vi "WSVCAP SHL Host TL Tester.vi"(0 "FPGA":T1) -> ()   [LabVIEW 2017]
uses:
  Type Defs/WSVCAP SHL DUT Number Enum.ctl
  <vilib>/userdefined/High Color/nirio_resource_hc.ctl
  Type Defs/WSVCAP SHL FPGA Enum.ctl
  Type Defs/WSVCAP SHL Tester System Cluster.ctl
  Type Defs/WSVCAP SHL I2C DUT Mask Mode Enum.ctl
panel:
  in  "Cap DAC":u8=144 caption="B Data In" format="0x%02x"
  in  "Set Cap DAC":bool
  in  "CP 35V":bool
  in  "CP 23.75V":bool
  in  "DVA On":bool
  in  "DVA Off":bool
  in  "CP 44V":bool
  in  "CP 40.25V":bool
  in  "Read Data DUT CMD":string caption="Read Data Out"
  in  "Read DUT":bool
  in  "CP On":bool
  in  "CP Off":bool
  in  "Write DUT":bool
  in  "Write Data DUT":string caption="Write Data Out"
  out "Read Data DUT Out":string caption="Data In"
  in  "Stop RFFE Cycle":bool
  in  "Start RFFE Cycle":bool
  in  "Command":string[](array[string])=["0703010F0F0F0F", "07030100000000"]
  in  "Post CMd Delay":dbl[](array[numeric])=[1.2e-05, 5.4e-05] min=0.0 max=0.5 format="%#.0p s"
  in  "Number of Commands":u32=2 min=1 max=4 step=1
  out "Cycle Count":u64=2 min=1 max=4 step=1
  in  "Monitor":bool
  out "AD7747 Values":string[][](table)
  in  "Mode":enum32{"All", "Single"}(radio)
  in  "RFFE Slave Address":u8=144 caption="Slave Address" format="0x%02x"
  out "Activity Log":string
  out "Simulate FPGA":bool
  out "Online":bool
  out "FPGA Resource":T2
  out "Status":string
  out "Busy":bool
  in  "I2C Bytes to Read":u8=1 caption="Bytes" min=1 max=4 step=1
  in  "Exit":bool
  out "Read Data I2C":u8[](array[numeric]) caption="Data In" format="0x%02x"
  in  "Read Reg I2C":u8 caption="Register" format="0x%02x"
  in  "Read I2C":bool
  in  "DUT":T3
  in  "Write Data I2C":u8 caption="Data Out" format="0x%02x"
  in  "Write Reg I2C":u8=144 caption="Register" format="0x%02x"
  in  "I2C Init":bool
  in  "Init Data":u8[](array[numeric])=[164, 160, 14, 33] caption="Data Out" format="0x%02x"
  in  "Init Reg":u8[](array[numeric])=[191, 7, 9, 10] caption="Register" format="0x%02x"
  in  "Write I2C":bool
  in  "I2C Slave Address":u8=144 caption="Slave Address" format="0x%02x"
  in  "RFFE Clock Rate (Hz)":dbl=1000000.0 caption="Clock Rate" format="%.1p Hz"
  in  "I2C Clock Rate (Hz)":dbl=100000.0 caption="Clock Rate" format="%.0p Hz"
  in  "Error":errorcluster
  # "WS1020 Tester"
  # "AD7747 (I2C)"
  # "C"
  # "DUT Control (RFFE)"
  # "DUT Cycling (RFFE)"
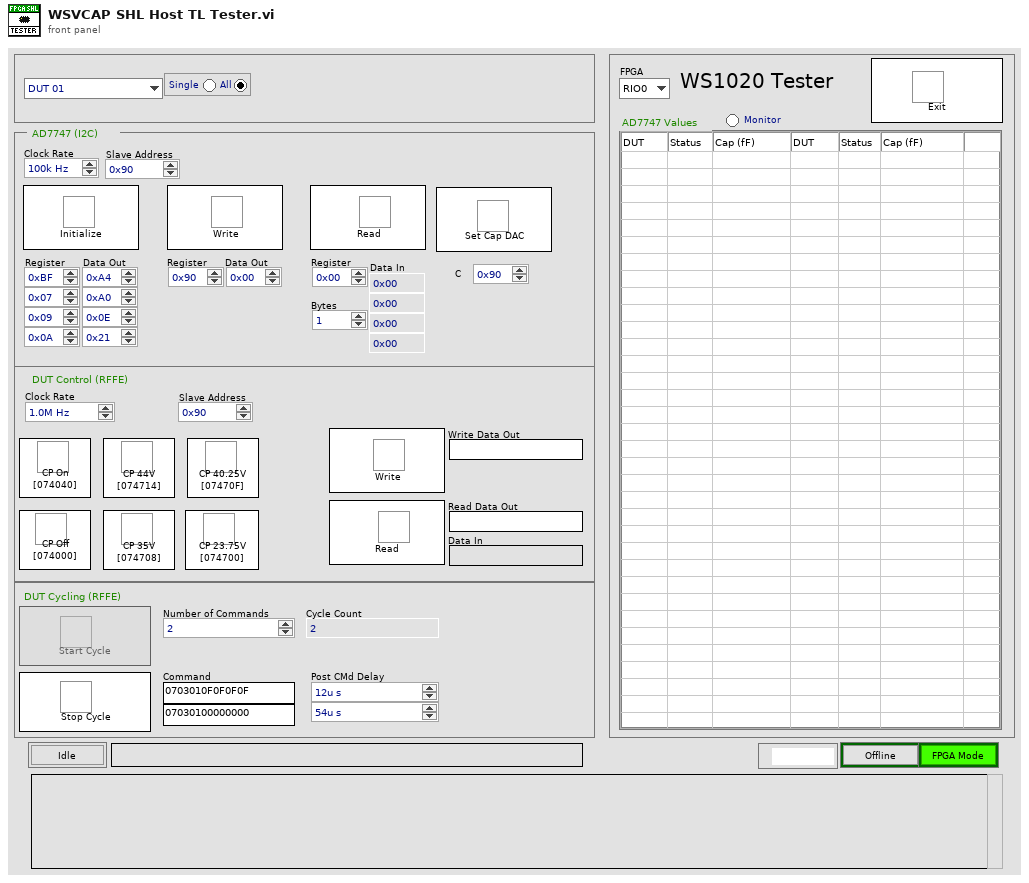
[diagram p1: front panel]
types:
  T1 = typedef "WSVCAP SHL FPGA Enum.ctl" = enum16{"RIO0", "RIO1"}
  T2 = typedef "nirio_resource_hc.ctl" = tag
  T3 = typedef "WSVCAP SHL DUT Number Enum.ctl" = enum16{"DUT 01", "DUT 02", "DUT 03", "DUT 04", "DUT 05", "DUT 06", "DUT 07", "DUT 08", "DUT 09", "DUT 10", "DUT 11", "DUT 12", "DUT 13", "DUT 14", "DUT 15", "DUT 16", "DUT 17", "DUT 18", "DUT 19", "DUT 20", "DUT 21", "DUT 22", "DUT 23", "DUT 24", "DUT 25", "DUT 26", "DUT 27", "DUT 28", "DUT 29", "DUT 30", "DUT 31", "DUT 32", "DUT 33", "DUT 34", "DUT 35", "DUT 36", "DUT 37", "DUT 38", "DUT 39", "DUT 40", "DUT 41", "DUT 42", "DUT 43", "DUT 44", "DUT 45", "DUT 46", "DUT 47", "DUT 48", "DUT 49", "DUT 50", "DUT 51", "DUT 52", "DUT 53", "DUT 54", "DUT 55", "DUT 56", "DUT 57", "DUT 58", "DUT 59", "DUT 60", "DUT 61", "DUT 62", "DUT 63", "DUT 64"}
  T4 = typedef "WSVCAP SHL Tester System Cluster.ctl" = cluster{"I2C Monitor":bool, "SPI Cyle":bool, "SPI Mode":enum32{"Write/Read", "Cycle"}, "RFFE Cyle":bool, "RFFE Mode":enum32{"Write/Read", "Cycle"}}
  T5 = typedef "WSVCAP SHL Core System Cluster.ctl" = cluster{"Settings":T6, "FPGA Resource":tag, "Online":bool, "I2C Wait Ticks":u32, "SPI Wait Ticks":u32, "RFFE Wait Ticks":u32, "FPGA VI Reference (FPGA Mode)":T7, "FPGA VI Reference (Sim Mode)":refnum<vi>}
  T6 = typedef "WSVCAP SHL I2C Settings Cluster.ctl" = cluster{"I2C Slave Address":u8, "I2C Clock Rate (Hz)":dbl, "SPI Clock Rate (Hz)":dbl, "RFFE Slave Address":u8, "RFFE Clock Rate (Hz)":dbl, "Simulate FPGA":bool, "C1 Cap DAC Default":u8, "C2 Cap DAC Default":u8, "C3 Cap DAC Default":u8, "C4 Cap DAC Default":u8}
  T7 = typedef "WSVCAP SHL FPGA Ref.ctl" = refnum<k20>
  T8 = enum8{"Enabled", "Disabled", "Disabled and Grayed Out"}
  T9 = typedef "WSVCAP SHL I2C DUT Mask Mode Enum.ctl" = enum16{"Custom", "All"}
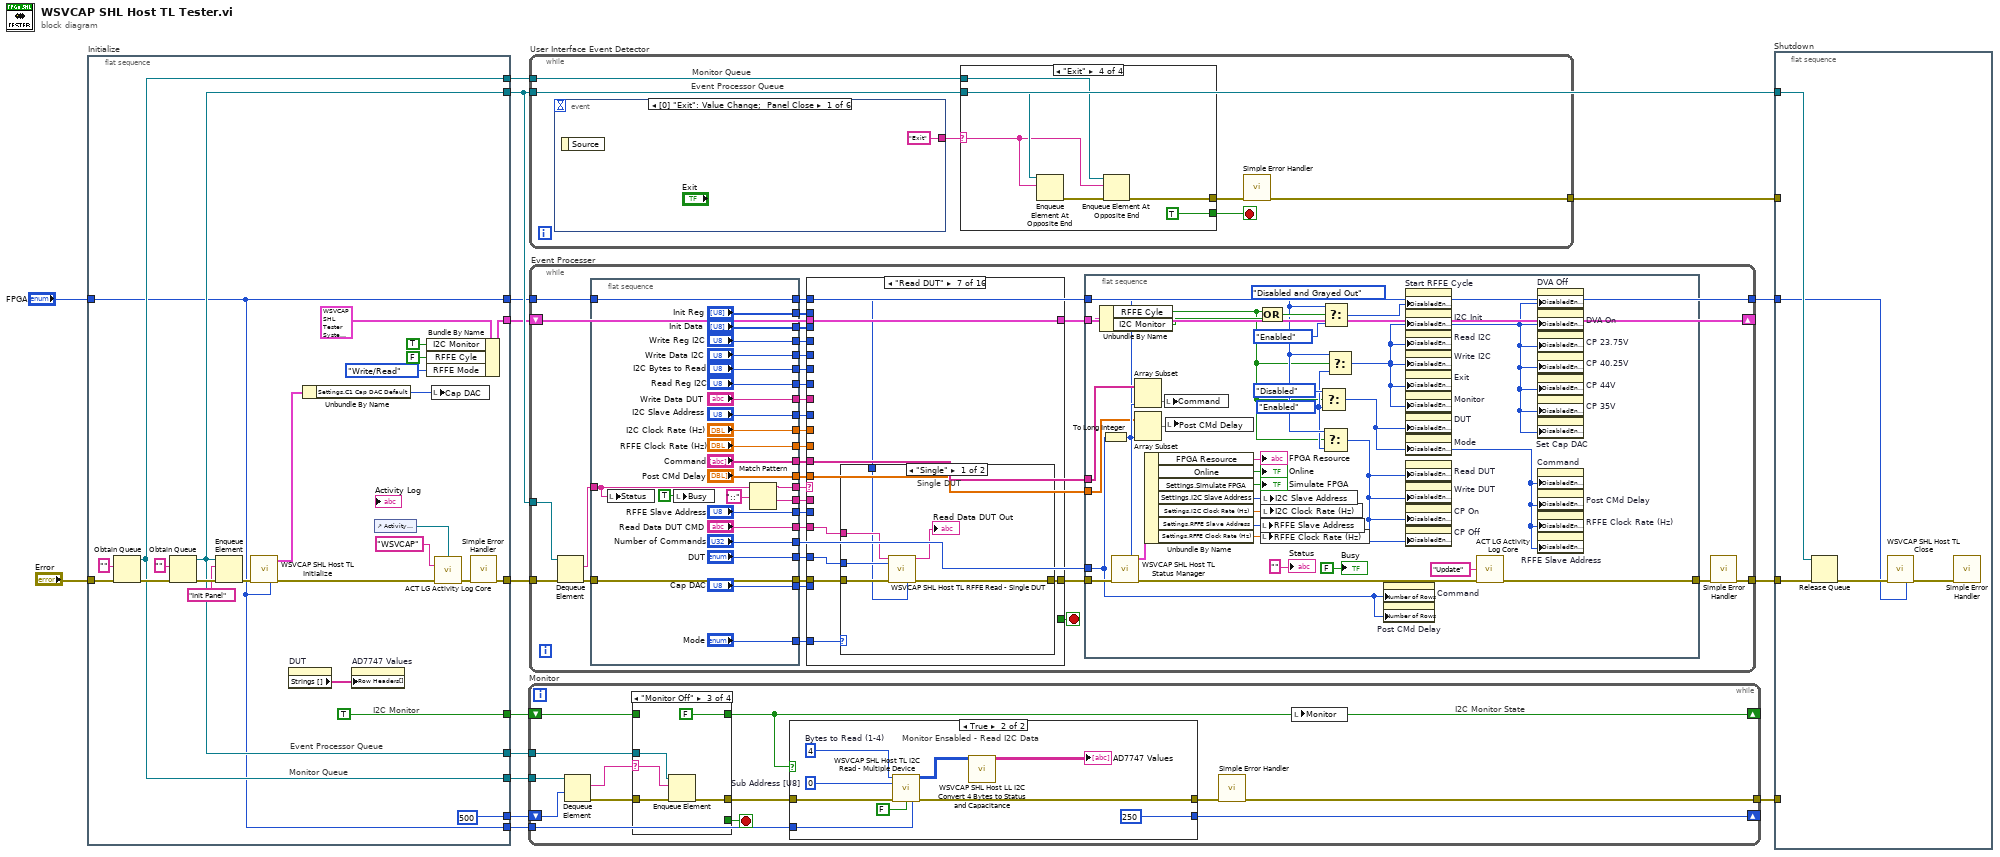
[diagram p0: block diagram]
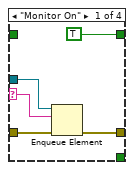
[diagram p2: hidden frame]
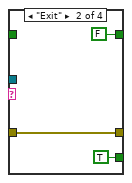
[diagram p3: hidden frame]
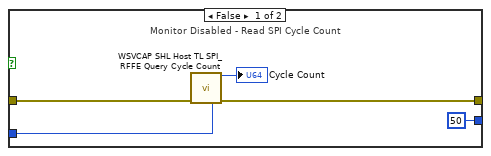
[diagram p5: hidden frame]
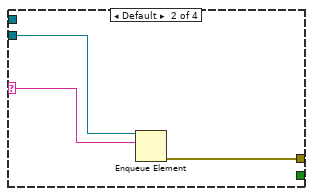
[diagram p7: hidden frame]
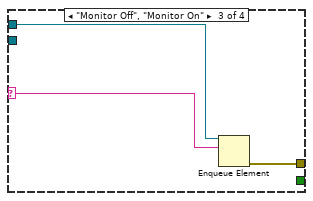
[diagram p8: hidden frame]
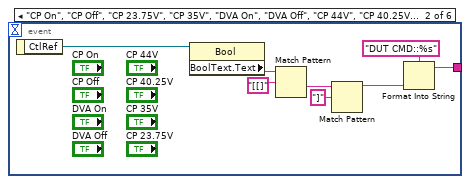
[diagram p9: hidden frame]
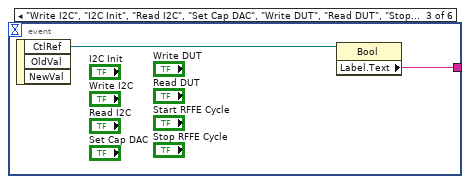
[diagram p10: hidden frame]
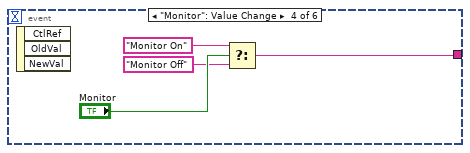
[diagram p11: hidden frame]
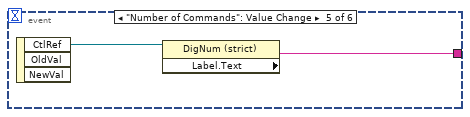
[diagram p12: hidden frame]
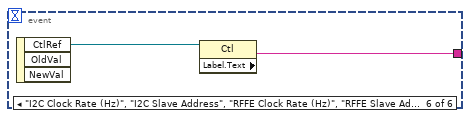
[diagram p13: hidden frame]
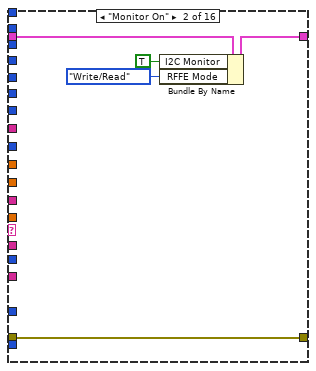
[diagram p15: hidden frame]
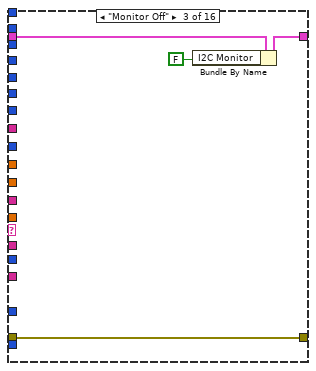
[diagram p16: hidden frame]
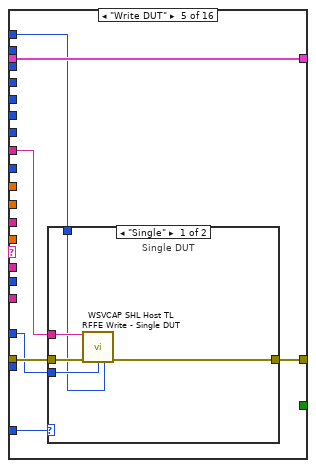
[diagram p18: hidden frame]
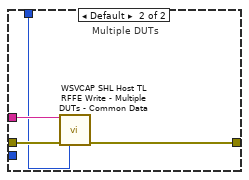
[diagram p19: hidden frame]
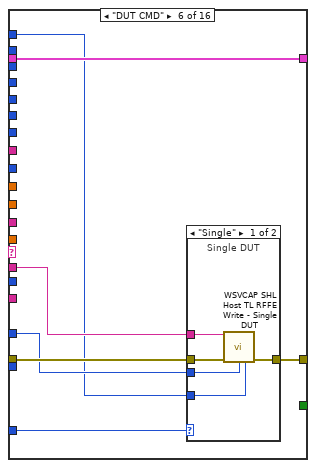
[diagram p20: hidden frame]
diagram:
  n1 = flat-sequence "Initialize" {
    tunnel: "Error" -> [w32]
    tunnel: [w30] -> w15
    tunnel: [TRUE ("Monitor")] -> w6
    tunnel: [w37] -> w11
    tunnel: [w28] -> w10
    tunnel: [w25] -> w9
    tunnel: [w30] -> w8
    tunnel: [w25] -> w7
    tunnel: [500 ("Wait Time (500ms)")] -> w5
    tunnel: "FPGA" -> [w17]
    tunnel: [w17] -> w3
    tunnel: [w17] -> w1
    frame #0 {
      # "I2C Monitor"
      # "Monitor Queue"
      # "Event Processor Queue"
      n2 = Obtain Queue(element data type="" ("name (unnamed)"), error in (no error)=w32) -> (queue out=w25:refnum<queue>, error out=w31:errorcluster)  [unwired: 3 in, 1 out]
      n3 = Obtain Queue(element data type="" ("name (unnamed)"), error in (no error)=w31) -> (queue out=w30:refnum<queue>, error out=w40:errorcluster)  [unwired: 3 in, 1 out]
      n4 = Enqueue Element(queue=w30, element="Init Panel" ("name (unnamed)"), error in (no error)=w40) -> (error out=w22:errorcluster)  [unwired: 1 in, 2 out]
      n5 = call "WSVCAP SHL Host TL Initialize.vi"("error in"=w22, "FPGA"=w17) -> ("System"=w20:T5, "error out"=w21:errorcluster)  [unwired: 12 in]
      n6 = property on="DUT" class="Enum (strict)"() -> ("Strings []"=w23:string[])  [unwired: 2 in, 2 out]
      n7 = Unbundle By Name(w20) -> ("Settings.C1 Cap DAC Default"=w19:u8)
      n8 = property on="AD7747 Values" class="Tbl (strict)"("Row Headers[]"=w23) -> ()  [unwired: 2 in, 2 out]
      n9 = control-ref of="Activity Log"() -> (w36:refnum<vi>)
      n10 = Bundle By Name(cluster=T4 {"I2C Monitor"=TRUE, "SPI Cyle"=TRUE, "SPI Mode"=enum."Write/Read", "RFFE Cyle"=FALSE, "RFFE Mode"=enum."Write/Read"}, "I2C Monitor"=TRUE, "RFFE Cyle"=FALSE ("I2C Monitor"), "RFFE Mode"=enum32{"Write/Read", "Cycle"}."Write/Read" ("SPI Mode")) -> (w28:T4)
      n11 = local write "Cap DAC"(w19) -> ()
      n12 = call "ACT LG Activity Log Core.vi"("Display Ref"=w36, "Source"="WSVCAP", "Error In (no error)"=w21) -> ("Error Out"=w38:errorcluster)  [unwired: 11 in, 1 out]
      n13 = call <vilib>:"Simple Error Handler.vi"("error in (no error)"=w38) -> ("error out"=w37:errorcluster)  [unwired: 4 in, 4 out]
    }
  }
  n14 = while "Monitor" {
    tunnel: [w46] -> w12
    shift-right: [w45] -> _
    shift-left: w6 -> [w52]
    tunnel: w9 -> [w50]
    tunnel: w8 -> [w49]
    shift-right: [w44] -> _
    shift-left: w5 -> [w43]
    tunnel: w1 -> [w42]
    stop <- w47 stop-if-true
    # "I2C Monitor State"
    n15 = Dequeue Element(queue=w50, timeout in ms (-1)=w43) -> (element=w53:string, error out=w51:errorcluster)  [unwired: 1 in, 2 out]
    n16 = case shown="\"Monitor Off\"" w53 {
      selector: w53 -> [w56 _ w64 _]
      tunnel: [TRUE FALSE FALSE w69] -> w45
      tunnel: w52 -> [_ _ _ w69]
      tunnel: w51 -> [w58 w61 w66 w68]
      tunnel: [w57 w61 w65 w68] -> w48
      tunnel: w49 -> [w55 _ w63 _]
      tunnel: [_ TRUE _ _] -> w47
      frame "Monitor On" {
        n17 = Enqueue Element(queue=w55, element=w56, error in (no error)=w58) -> (error out=w57:errorcluster)  [unwired: 1 in, 2 out]
      }
      frame "Exit" {
      }
      frame "Monitor Off" {
        n18 = Enqueue Element(queue=w63, element=w64, error in (no error)=w66) -> (error out=w65:errorcluster)  [unwired: 1 in, 2 out]
      }
      frame Default {
      }
    }
    n19 = case shown="True" w45 {
      tunnel: [w72 w78] -> w54
      tunnel: w48 -> [w73 w79]
      tunnel: [50 ("Wait Time (500ms)") 250 ("Wait Time (500ms)")] -> w44
      tunnel: w42 -> [w70 w75]
      frame False {
        # "Monitor Disabled - Read SPI Cycle Count"
        n20 = call "WSVCAP SHL Host TL SPI_RFFE Query Cycle Count.vi"("error in"=w73, "FPGA"=w70) -> ("Cycle Count"=→"Cycle Count":u64, "error out"=w72:errorcluster)  [unwired: 12 in]
      }
      frame True {
        w82 = u8 4  # Bytes to Read (1-4)
        w83 = u8 0  # Sub Address [U8]
        # "Monitor Ensabled - Read I2C Data"
        n21 = call "WSVCAP SHL Host TL I2C Read - Multiple Device.vi"("Bytes to Read (1-4)"=w82, "Sub Address [U8]"=w83, "error in"=w79, "Log (T)"=FALSE, "FPGA"=w75) -> ("C:1-64 Read Data [U8]"=w81:u8[][], "error out"=w78:errorcluster)  [unwired: 9 in]
        n22 = call "WSVCAP SHL Host LL I2C Convert 4 Bytes to Status and Capacitance.vi"("C:1-64 Read Data [U8]"=w81) -> ("AD7747 Values"=→"AD7747 Values":string[][])  [unwired: 14 in]
      }
    }
    n23 = call <vilib>:"Simple Error Handler.vi"("error in (no error)"=w54) -> ("error out"=w46:errorcluster)  [unwired: 4 in, 4 out]
    n24 = local write "Monitor"(w45) -> ()
  }
  n25 = while "User Interface Event Detector" {
    tunnel: w15 -> [w88]
    tunnel: [w85] -> w13
    tunnel: w7 -> [w84]
    stop <- w86 stop-if-true
    # "Monitor Queue"
    # "Event Processor Queue"
    n26 = event shown="[0] \"Exit\": Value Change;  Panel Close" {
      selector: _ -> [_ _ _ _ _ _]
      dyn-events: _ -> [_ _ _ _ _ _]
      timeout: _ -> [_ _ _ _ _ _]
      tunnel: ["Exit" ("Label.Text") w109 w112 w113 w118 w120] -> w89
      event "Exit": Value Change; Panel Close {
        n27 = event-data() -> ()  [unwired: 1 in, 1 out]
      }
      event "CP On", "CP Off", "CP 23.75V", "CP 35V", "DVA On", "DVA Off", "CP 44V", "CP 40.25V": Value Change {
        n28 = event-data() -> ("CtlRef"=w110:refnum<vi>)  [unwired: 1 in]
        n29 = property class="Bool"(reference=w110) -> ("BoolText.Text"=w107:string)  [unwired: 1 in, 2 out]
        n30 = Match Pattern(string=w107, regular expression="[[]") -> (after substring=w105:string)  [unwired: 1 in, 3 out]
        n31 = Match Pattern(string=w105, regular expression="]") -> (before substring=w103:string)  [unwired: 1 in, 3 out]
        n32 = Format Into String(format string="DUT CMD::%s", w103) -> (resulting string=w109:string)  [unwired: 2 in, 1 out]
      }
      event "Write I2C", "I2C Init", "Read I2C", "Set Cap DAC", "Write DUT", "Read DUT", "Stop RFFE Cycle", "Start RFFE Cycle": Value Change {
        n33 = event-data() -> ("CtlRef"=w111:refnum<vi>)  [unwired: 1 in, 2 out]
        n34 = property class="Bool"(reference=w111) -> ("Label.Text"=w112:string)  [unwired: 1 in, 2 out]
      }
      event "Monitor": Value Change {
        n35 = event-data() -> ()  [unwired: 1 in, 3 out]
        n36 = Select(t="Monitor On" ("Label.Text"), s="Monitor", f="Monitor Off" ("Label.Text")) -> (s? t:f=w113:string)
      }
      event "Number of Commands": Value Change {
        n37 = event-data() -> ("CtlRef"=w117:refnum<vi>)  [unwired: 1 in, 2 out]
        n38 = property class="DigNum (strict)"(reference=w117) -> ("Label.Text"=w118:string)  [unwired: 1 in, 2 out]
      }
      event "I2C Clock Rate (Hz)", "I2C Slave Address", "RFFE Clock Rate (Hz)", "RFFE Slave Address", "Mode": Value Change {
        n39 = event-data() -> ("CtlRef"=w119:refnum<vi>)  [unwired: 1 in, 2 out]
        n40 = property class="Ctl"(reference=w119) -> ("Label.Text"=w120:string)  [unwired: 1 in, 2 out]
      }
    }
    n41 = case shown="\"Exit\"" w89 {
      selector: w89 -> [_ w92 w95 w96]
      tunnel: w88 -> [_ w91 _ w101]
      tunnel: [_ w90 w94 w98] -> w87
      tunnel: [_ _ _ TRUE] -> w86
      tunnel: w84 -> [_ _ w93 w97]
      frame "" {
      }
      frame Default {
        n42 = Enqueue Element(queue=w91, element=w92) -> (error out=w90:errorcluster)  [unwired: 2 in, 2 out]
      }
      frame "Monitor Off", "Monitor On" {
        n43 = Enqueue Element(queue=w93, element=w95) -> (error out=w94:errorcluster)  [unwired: 2 in, 2 out]
      }
      frame "Exit" {
        n44 = Enqueue Element At Opposite End(queue=w101, element=w96) -> (error out=w99:errorcluster)  [unwired: 2 in, 2 out]
        n45 = Enqueue Element At Opposite End(queue=w97, element=w96, error in (no error)=w99) -> (error out=w98:errorcluster)  [unwired: 1 in, 2 out]
      }
    }
    n46 = call <vilib>:"Simple Error Handler.vi"("error in (no error)"=w87) -> ("error out"=w85:errorcluster)  [unwired: 4 in, 4 out]
  }
  n47 = while "Event Processer" {
    tunnel: w15 -> [w153]
    tunnel: [w151] -> w14
    tunnel: w11 -> [w133]
    shift-right: [w128] -> _
    shift-left: w10 -> [w129]
    tunnel: w3 -> [w121]
    tunnel: [w121] -> w2
    stop <- w152 stop-if-true
    n48 = Dequeue Element(queue=w153, error in (no error)=w133) -> (element=w149:string, error out=w147:errorcluster)  [unwired: 1 in, 2 out]
    n49 = flat-sequence {
      tunnel: ["I2C Clock Rate (Hz)"] -> w150
      tunnel: [w191] -> w148
      tunnel: w149 -> [w192]
      tunnel: [w210] -> w146
      tunnel: w147 -> [w210]
      tunnel: ["I2C Bytes to Read"] -> w145
      tunnel: ["I2C Slave Address"] -> w144
      tunnel: ["RFFE Clock Rate (Hz)"] -> w143
      tunnel: ["DUT"] -> w140
      tunnel: ["Init Data"] -> w139
      tunnel: ["Init Reg"] -> w138
      tunnel: ["Write Reg I2C"] -> w137
      tunnel: ["Write Data I2C"] -> w136
      tunnel: ["Read Reg I2C"] -> w135
      tunnel: ["Write Data DUT"] -> w134
      tunnel: ["Mode"] -> w125
      tunnel: ["Command"] -> w131
      tunnel: ["Post CMd Delay"] -> w130
      tunnel: ["Number of Commands"] -> w132
      tunnel: ["RFFE Slave Address"] -> w127
      tunnel: ["Read Data DUT CMD"] -> w126
      tunnel: [w189] -> w124
      tunnel: ["Cap DAC"] -> w123
      tunnel: [w187] -> w122
      tunnel: w121 -> [w187]
      frame #0 {
        n50 = local write "Status"(w192) -> ()
        n51 = local write "Busy"(TRUE ("Busy")) -> ()
        n52 = Match Pattern(string=w192, regular expression="::") -> (before substring=w191:string, after substring=w189:string)  [unwired: 1 in, 2 out]
      }
    }
    n53 = case shown="\"Read DUT\"" w148 {
      tunnel: w146 -> [w213 w218 w222 w224 w231 w247 w263 w288 w305 w313 w334 w344 w374 w376 w383 w389]
      tunnel: [w213 w218 w222 w224 w230 w246 w262 w287 w304 w312 w333 w343 w369 w376 w380 w387] -> w142
      tunnel: [_ _ _ _ _ _ _ _ _ _ _ _ _ TRUE _ _] -> w152
      tunnel: w150 -> [_ _ _ _ _ _ _ _ _ _ _ _ _ _ w382 _]
      tunnel: w145 -> [_ _ _ _ _ _ _ _ _ _ _ _ w371 _ _ _]
      tunnel: w144 -> [_ _ _ _ _ _ _ _ _ _ _ _ _ _ w381 _]
      tunnel: w143 -> [_ _ _ _ _ _ _ _ _ _ _ _ _ _ _ w388]
      tunnel: w140 -> [_ _ _ _ w228 w244 w260 w285 _ w310 _ w341 w373 _ _ _]
      tunnel: w139 -> [_ _ _ _ _ _ _ _ _ _ _ w339 _ _ _ _]
      tunnel: w138 -> [_ _ _ _ _ _ _ _ _ _ _ w340 _ _ _ _]
      tunnel: w137 -> [_ _ _ _ _ _ _ _ _ w309 _ _ _ _ _ _]
      tunnel: w136 -> [_ _ _ _ _ _ _ _ _ w308 _ _ _ _ _ _]
      tunnel: w135 -> [_ _ _ _ _ _ _ _ _ _ _ _ w372 _ _ _]
      tunnel: w134 -> [_ _ _ _ w227 _ _ _ _ _ _ _ _ _ _ _]
      tunnel: w125 -> [_ _ _ _ w229 w245 w261 w286 _ w311 _ w342 _ _ _ _]
      tunnel: w131 -> [_ _ _ _ _ _ _ w284 _ _ _ _ _ _ _ _]
      tunnel: w130 -> [_ _ _ _ _ _ _ w283 _ _ _ _ _ _ _ _]
      tunnel: [w212 w216 w220 w223 w226 w243 w259 w281 w301 w307 w336 w338 w368 w375 w379 w386] -> w128
      tunnel: w129 -> [w212 w217 w221 w223 w226 w243 w259 w282 w302 w307 w336 w338 w368 w375 w379 w386]
      tunnel: w127 -> [_ _ _ _ _ _ _ _ _ _ _ _ _ _ _ w385]
      tunnel: w126 -> [_ _ _ _ _ _ w258 _ _ _ _ _ _ _ _ _]
      tunnel: w124 -> [_ _ _ _ _ w242 _ _ _ _ _ _ _ _ _ _]
      tunnel: w123 -> [_ _ _ _ _ _ _ w279 _ _ w332 _ _ _ _ _]
      tunnel: w122 -> [_ _ _ _ w225 w241 w257 w278 w300 w306 w331 w337 w367 _ w378 w384]
      frame Default {
      }
      frame "Monitor On" {
        n54 = Bundle By Name(cluster=w217, "I2C Monitor"=TRUE, "RFFE Mode"=enum32{"Write/Read", "Cycle"}."Write/Read" ("SPI Mode")) -> (w216:T4)
      }
      frame "Monitor Off" {
        n55 = Bundle By Name(cluster=w221, "I2C Monitor"=FALSE) -> (w220:T4)
      }
      frame "Number of Commands" {
      }
      frame "Write DUT" {
        n56 = case shown="\"Single\"" w229 {
          tunnel: w231 -> [w236 w240]
          tunnel: [w233 w239] -> w230
          tunnel: w228 -> [w234 _]
          tunnel: w227 -> [w235 w238]
          tunnel: w225 -> [w232 w237]
          frame "Single" {
            # "Single DUT"
            n57 = call "WSVCAP SHL Host TL RFFE Write - Single DUT.vi"("Data Out"=w235, "error in"=w236, "DUT"=w234, "FPGA"=w232) -> ("error out"=w233:errorcluster)  [unwired: 11 in]
          }
          frame Default {
            # "Multiple DUTs"
            n58 = call "WSVCAP SHL Host TL RFFE Write - Multiple DUTs - Common Data.vi"("Data Out"=w238, "error in"=w240, "FPGA"=w237) -> ("error out"=w239:errorcluster)  [unwired: 12 in]
          }
        }
      }
      frame "DUT CMD" {
        n59 = case shown="\"Single\"" w245 {
          tunnel: w247 -> [w252 w256]
          tunnel: [w249 w255] -> w246
          tunnel: w244 -> [w250 _]
          tunnel: w242 -> [w251 w254]
          tunnel: w241 -> [w248 w253]
          frame "Single" {
            # "Single DUT"
            n60 = call "WSVCAP SHL Host TL RFFE Write - Single DUT.vi"("Data Out"=w251, "error in"=w252, "DUT"=w250, "FPGA"=w248) -> ("error out"=w249:errorcluster)  [unwired: 11 in]
          }
          frame Default {
            # "Multiple DUTs"
            n61 = call "WSVCAP SHL Host TL RFFE Write - Multiple DUTs - Common Data.vi"("Data Out"=w254, "error in"=w256, "FPGA"=w253) -> ("error out"=w255:errorcluster)  [unwired: 12 in]
          }
        }
      }
      frame "Read DUT" {
        n62 = case shown="\"Single\"" w261 {
          tunnel: w263 -> [w269 w277]
          tunnel: [w267 w276] -> w262
          tunnel: w260 -> [w268 w273]
          tunnel: w258 -> [w265 w275]
          tunnel: w257 -> [w264 w270]
          frame "Single" {
            # "Single DUT"
            n63 = call "WSVCAP SHL Host TL RFFE Read - Single DUT.vi"("Data Out"=w265, "error in"=w269, "DUT"=w268, "FPGA"=w264) -> ("Data In"=→"Read Data DUT Out":string, "error out"=w267:errorcluster)  [unwired: 10 in]
          }
          frame Default {
            # "Multiple DUTs"
            n64 = To Long Integer(number=w273) -> (32bit integer=w272:i32)
            n65 = call "WSVCAP SHL Host TL RFFE Read - Multiple DUTs - Common Data.vi"("Data Out"=w275, "error in"=w277, "FPGA"=w270) -> ("RFFE Data In"=w274:string[], "error out"=w276:errorcluster)  [unwired: 11 in]
            n66 = Index Array(array=w274, index=w272) -> (element=w271:string)
            n67 = local write "Read Data DUT Out"(w271) -> ()
          }
        }
      }
      frame "Start RFFE Cycle" {
        n68 = case shown="\"All\"" w286 {
          tunnel: w288 -> [w294 w299]
          tunnel: [w293 w298] -> w287
          tunnel: w285 -> [w292 _]
          tunnel: w284 -> [w291 w297]
          tunnel: w283 -> [w290 w296]
          tunnel: w279 -> [_ _]
          tunnel: w278 -> [w289 w295]
          frame Default {
            # "Single DUT"
            n69 = call "WSVCAP SHL Host TL RFFE Write Cycle - Single DUT.vi"("Data Out (Cycle Commands)"=w291, "Post Command Delay"=w290, "error in"=w294, "DUT"=w292, "FPGA"=w289) -> ("error out"=w293:errorcluster)  [unwired: 10 in]
          }
          frame "All" {
            # "Multiple DUTs"
            n70 = call "WSVCAP SHL Host TL RFFE Write Cycle - Multiple DUTs - Common Data.vi"("Data Out (Cycle Commands)"=w297, "Post Command Delay"=w296, "error in"=w299, "FPGA"=w295) -> ("error out"=w298:errorcluster)  [unwired: 11 in]
          }
        }
        n71 = Bundle By Name(cluster=w282, "RFFE Cyle"=TRUE ("SPI Cyle")) -> (w281:T4)
      }
      frame "Stop RFFE Cycle" {
        n72 = call "WSVCAP SHL Host TL RFFE Stop Write Cycle.vi"("error in"=w305, "FPGA"=w300) -> ("error out"=w304:errorcluster)  [unwired: 13 in]
        n73 = Bundle By Name(cluster=w302, "RFFE Cyle"=FALSE ("SPI Cyle")) -> (w301:T4)
      }
      frame "Write I2C" {
        n74 = case shown="Default" w311 {
          selector: w311 -> [_ w324]
          tunnel: w313 -> [w319 w328]
          tunnel: [w318 w327] -> w312
          tunnel: w310 -> [w317 _]
          tunnel: w309 -> [w316 w326]
          tunnel: w308 -> [w315 w325]
          tunnel: w306 -> [w314 w320]
          frame "Single" {
            # "Single DUT"
            n75 = call "WSVCAP SHL Host TL I2C Write - Single Device.vi"("Sub Address [U8]"=w316, "FPGA"=w314, "Data Out [U8]"=w315, "error in"=w319, "DUT"=w317) -> ("error out"=w318:errorcluster)  [unwired: 10 in]
          }
          frame Default {
            # "Multiple DUTs"
            n76 = Format Into String(w324) -> (resulting string=w323:string)  [unwired: 3 in, 1 out]
            n77 = Scan From String(input string=w323, default 1=WSVCAP_SHL_I2C_DUT_Mask_Mode_Enum."All" ("DUT Mask Mode (All)")) -> (output 1=w321:T9)  [unwired: 3 in, 3 out]
            n78 = call "WSVCAP SHL Host TL I2C Write - Multiple Device - Common Data.vi"("Sub Address"=w326, "FPGA"=w320, "Data Out [U8]"=w325, "error in"=w328, "DUT Mask Mode (All)"=w321) -> ("error out"=w327:errorcluster)  [unwired: 10 in]
          }
        }
      }
      frame "Set Cap DAC" {
        n79 = Initialize Array(w332, 64 ("dimension size")) -> (w335:u8[])
        n80 = call "WSVCAP SHL Host TL I2C Write - Multiple Device - Unique Data.vi"("C1 Data"=w335, "Sub Address"=u8 11, "FPGA"=w331, "error in"=w334) -> ("error out"=w333:errorcluster)  [unwired: 11 in]
      }
      frame "I2C Init" {
        n81 = for {
          tunnel: w342 -> [w349]
          tunnel: w341 -> [w348]
          tunnel: w340 -> [w347] mode=indexing
          tunnel: w339 -> [w346] mode=indexing
          shift-right: [w350] -> w343
          shift-left: w344 -> [w351]
          tunnel: w337 -> [w345]
          n82 = case shown="\"Single\"" w349 {
            selector: w349 -> [_ w360]
            tunnel: w351 -> [w357 w366]
            tunnel: [w356 w365] -> w350
            tunnel: w348 -> [w355 _]
            tunnel: w347 -> [w354 w364]
            tunnel: w346 -> [w353 w363]
            tunnel: w345 -> [w352 w358]
            frame "Single" {
              # "Single DUT"
              n83 = call "WSVCAP SHL Host TL I2C Write - Single Device.vi"("Sub Address [U8]"=w354, "FPGA"=w352, "Data Out [U8]"=w353, "error in"=w357, "DUT"=w355) -> ("error out"=w356:errorcluster)  [unwired: 10 in]
            }
            frame Default {
              # "Multiple DUTs"
              n84 = Format Into String(w360) -> (resulting string=w362:string)  [unwired: 3 in, 1 out]
              n85 = Scan From String(input string=w362, default 1=WSVCAP_SHL_I2C_DUT_Mask_Mode_Enum."All" ("DUT Mask Mode (All)")) -> (output 1=w359:T9)  [unwired: 3 in, 3 out]
              n86 = call "WSVCAP SHL Host TL I2C Write - Multiple Device - Common Data.vi"("Sub Address"=w364, "FPGA"=w358, "Data Out [U8]"=w363, "error in"=w366, "DUT Mask Mode (All)"=w359) -> ("error out"=w365:errorcluster)  [unwired: 10 in]
            }
          }
        }
      }
      frame "Read I2C" {
        n87 = call "WSVCAP SHL Host TL I2C Read - Single Device.vi"("Bytes to Read (1-4)"=w371, "FPGA"=w367, "Sub Address [U8]"=w372, "error in"=w374, "DUT"=w373) -> ("Device Data"=→"Read Data I2C":u8[], "error out"=w369:errorcluster)  [unwired: 9 in]
      }
      frame "Exit" {
      }
      frame "I2C Clock Rate (Hz)", "I2C Slave Address" {
        n88 = call "WSVCAP SHL Host TL I2C Configure.vi"("I2C_Slave Address"=w381, "Clock Rate (Hz)"=w382, "error in"=w383, "FPGA"=w378) -> ("error out"=w380:errorcluster)  [unwired: 10 in, 1 out]
      }
      frame "RFFE Clock Rate (Hz)", "RFFE Slave Address" {
        n89 = call "WSVCAP SHL Host TL RFFE Configure.vi"("RFFE Slave Address"=w385, "Clock Rate (Hz)"=w388, "error in"=w389, "FPGA"=w384) -> ("error out"=w387:errorcluster)  [unwired: 10 in, 1 out]
      }
    }
    n90 = flat-sequence {
      tunnel: [w174] -> w141
      tunnel: w142 -> [w184]
      tunnel: w132 -> [w173]
      tunnel: w131 -> [w171]
      tunnel: w130 -> [w169]
      tunnel: w128 -> [w167]
      tunnel: w121 -> [w154]
      frame #0 {
        w161 = T8."Enabled" ("Disabled")
        w162 = T8."Disabled and Grayed Out" ("Disabled")
        n91 = Unbundle By Name(w167) -> ("RFFE Cyle"=w160:bool, "I2C Monitor"=w166:bool)
        n92 = To Long Integer(number=w173) -> (32bit integer=w172:i32)
        n93 = call "WSVCAP SHL Host TL Status Manager.vi"("error in"=w184, "FPGA"=w154) -> ("System Out"=w183:T5, "error out"=w176:errorcluster)  [unwired: 12 in]
        n94 = Array Subset(array=w171, length=w172) -> (w170:string[])  [unwired: 1 in]
        n95 = Array Subset(array=w169, length=w172) -> (w168:dbl[])  [unwired: 1 in]
        n96 = Unbundle By Name(w183) -> ("FPGA Resource"=→"FPGA Resource":tag, "Online"=→"Online":bool, "Settings.Simulate FPGA"=→"Simulate FPGA":bool, "Settings.I2C Slave Address"=w182:u8, "Settings.I2C Clock Rate (Hz)"=w181:dbl, "Settings.RFFE Slave Address"=w158:u8, "Settings.RFFE Clock Rate (Hz)"=w180:dbl)
        n97 = local write "Command"(w170) -> ()
        n98 = local write "Post CMd Delay"(w168) -> ()
        n99 = local write "RFFE Slave Address"(w158) -> ()
        n100 = local write "RFFE Clock Rate (Hz)"(w180) -> ()
        n101 = local write "I2C Slave Address"(w182) -> ()
        n102 = local write "I2C Clock Rate (Hz)"(w181) -> ()
        n103 = Compound Arithmetic op=OR(w160, w166) -> (w163:bool)
        n104 = Select(t=T8."Disabled" ("Disabled"), s=w160, f=w161) -> (s? t:f=w157:T8)
        n105 = Select(t=w162, s=w160, f=w161) -> (s? t:f=w155:T8)
        n106 = Select(t=w162, s=w163, f=T8."Enabled" ("Disabled")) -> (s? t:f=w159:T8)
        n107 = Select(t=w162, s=w160, f=w161) -> (s? t:f=w156:T8)
        n108 = property on="Command" class="Arr (strict)"("Number of Rows"=w173) -> ()  [unwired: 2 in, 2 out]
        n109 = property on="Post CMd Delay" class="Arr (strict)"("Number of Rows"=w173) -> ()  [unwired: 2 in, 2 out]
        n110 = property on="Start RFFE Cycle" class="Bool"("DisabledEnum"=w159) -> ()  [unwired: 2 in, 2 out]
        n111 = property on="I2C Init" class="Bool"("DisabledEnum"=w156) -> ()  [unwired: 2 in, 2 out]
        n112 = property on="Read I2C" class="Bool"("DisabledEnum"=w156) -> ()  [unwired: 2 in, 2 out]
        n113 = property on="Write I2C" class="Bool"("DisabledEnum"=w156) -> ()  [unwired: 2 in, 2 out]
        n114 = property on="Exit" class="Bool"("DisabledEnum"=w156) -> ()  [unwired: 2 in, 2 out]
        n115 = property on="Monitor" class="Bool (strict)"("DisabledEnum"=w156) -> ()  [unwired: 2 in, 2 out]
        n116 = property on="DUT" class="Enum (strict)"("DisabledEnum"=w157) -> ()  [unwired: 2 in, 2 out]
        n117 = property on="Mode" class="RadioBtnsControl (strict)"("DisabledEnum"=w157) -> ()  [unwired: 2 in, 2 out]
        n118 = property on="Read DUT" class="Bool"("DisabledEnum"=w155) -> ()  [unwired: 2 in, 2 out]
        n119 = property on="Write DUT" class="Bool"("DisabledEnum"=w155) -> ()  [unwired: 2 in, 2 out]
        n120 = property on="CP On" class="Bool"("DisabledEnum"=w155) -> ()  [unwired: 2 in, 2 out]
        n121 = property on="CP Off" class="Bool"("DisabledEnum"=w155) -> ()  [unwired: 2 in, 2 out]
        n122 = call "ACT LG Activity Log Core.vi"("Log Line"="Update", "Error In (no error)"=w176) -> ("Error Out"=w174:errorcluster)  [unwired: 12 in, 1 out]
        n123 = property on="DVA Off" class="Bool"("DisabledEnum"=w156) -> ()  [unwired: 2 in, 2 out]
        n124 = property on="DVA On" class="Bool"("DisabledEnum"=w156) -> ()  [unwired: 2 in, 2 out]
        n125 = property on="CP 23.75V" class="Bool"("DisabledEnum"=w156) -> ()  [unwired: 2 in, 2 out]
        n126 = property on="CP 40.25V" class="Bool"("DisabledEnum"=w156) -> ()  [unwired: 2 in, 2 out]
        n127 = property on="CP 44V" class="Bool"("DisabledEnum"=w156) -> ()  [unwired: 2 in, 2 out]
        n128 = property on="CP 35V" class="Bool"("DisabledEnum"=w156) -> ()  [unwired: 2 in, 2 out]
        n129 = property on="Set Cap DAC" class="Bool"("DisabledEnum"=w156) -> ()  [unwired: 2 in, 2 out]
        n130 = property on="Command" class="Arr (strict)"("DisabledEnum"=w157) -> ()  [unwired: 2 in, 2 out]
        n131 = property on="Post CMd Delay" class="Arr (strict)"("DisabledEnum"=w157) -> ()  [unwired: 2 in, 2 out]
        n132 = property on="RFFE Clock Rate (Hz)" class="DigNum (strict)"("DisabledEnum"=w157) -> ()  [unwired: 2 in, 2 out]
        n133 = property on="RFFE Slave Address" class="DigNum (strict)"("DisabledEnum"=w157) -> ()  [unwired: 2 in, 2 out]
        "Busy" <- FALSE ("Busy")
        "Status" <- "" ("Status")
      }
    }
    n134 = call <vilib>:"Simple Error Handler.vi"("error in (no error)"=w141) -> ("error out"=w151:errorcluster)  [unwired: 4 in, 4 out]
  }
  n135 = flat-sequence "Shutdown" {
    tunnel: w15 -> [w394]
    tunnel: w14 -> [w393]
    tunnel: w13 -> [_]
    tunnel: w12 -> [_]
    tunnel: w2 -> [w390]
    frame #0 {
      n136 = Release Queue(queue=w394, error in (no error)=w393) -> (error out=w392:errorcluster)  [unwired: 1 in, 2 out]
      n137 = call "WSVCAP SHL Host TL Close.vi"("error in"=w392, "FPGA"=w390) -> ("error out"=w391:errorcluster)  [unwired: 13 in]
      n138 = call <vilib>:"Simple Error Handler.vi"("error in (no error)"=w391) -> ()  [unwired: 4 in, 5 out]
    }
  }
